vi "Untitled 5.vi"() -> ()   [LabVIEW 2015]
uses:
  <vilib>/Utility/Data Type/Type Definitions/Data Type.ctl
  <vilib>/Utility/Data Type/Type Definitions/Memory Info.ctl
  <vilib>/Utility/Data Type/Type Definitions/Memory Type.ctl
  <vilib>/Utility/Data Type/Type Definitions/Type Definition Info.ctl
  <vilib>/addons/msgpack/msgpack.lvlib
  <vilib>/Utility/Data Type/NI_Data Type.lvlib
  msgpackalt.dll
panel:
  out "dimension size":i32=3
  out "unsigned byte array 3":u8[](array[numeric]) format="%x"
  out "Type Definition Info":T1
  out "Array Lengths":T2[](array[typedef])
  out "Type 2":T4
  out "Type":T4
  out "data string 2":string
  out "Size(s)":u32[](array[numeric]) format="%x"
  out "data string":string
  out "unsigned byte array 2":u8[](array[numeric])
  out "unsigned byte array":u8[](array[numeric]) format="%x"
  out "size(s) 2":i32
  out "size(s)":i32 format="%x"
  out "data 2":variant[][][](array[variant])
  out "x-y":u32
  out "x = y?":bool
  out "data":string
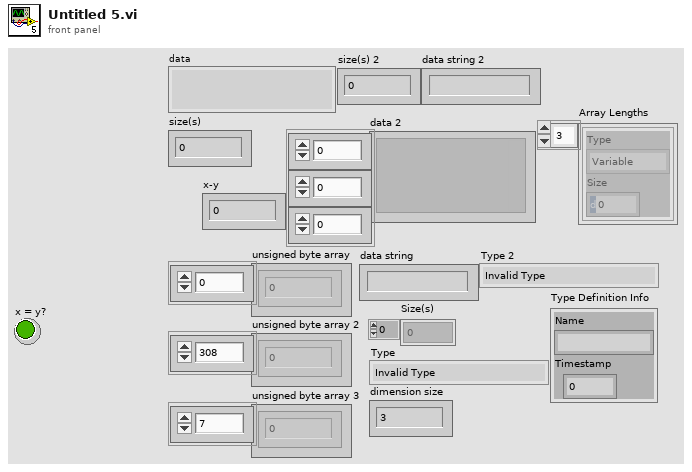
[diagram p1: front panel]
types:
  T1 = typedef "NI_Data Type.lvlib/Type Definition Info.ctl" = cluster{"Name":string, "Timestamp":u32}
  T2 = typedef "NI_Data Type.lvlib/Memory Info.ctl" = cluster{"Type":T3, "Size":u32}
  T3 = typedef "NI_Data Type.lvlib/Memory Type.ctl" = enum16{"Variable", "Fixed", "Bounded"}
  T4 = typedef "NI_Data Type.lvlib/Data Type.ctl" = enum8{"Invalid Type", "Void", "I8", "I16", "I32", "I64", "U8", "U16", "U32", "U64", "Single Float", "Double Float", "Extended Float", "Single Complex", "Double Complex", "Extended Complex", "Enum U8", "Enum U16", "Enum U32", "Enum U64", "Single Float With Unit", "Double Float With Unit", "Extended Float With Unit", "Single Complex with Unit", "Double Complex with Unit", "Extended Complex with Unit", "Boolean", "String", "Path", "Picture", "Tag", "Array", "Cluster", "Variant", "LV Variant", "Waveform", "Timestamp", "Digital Waveform", "Digital Data", "ExpressData", "Refnum", "External Data", "VI", "Poly VI", "LabVIEW Class Instance", "Fixed Point"}
  T5 = enum16{"big-endian, network order", "native, host order", "little-endian"}
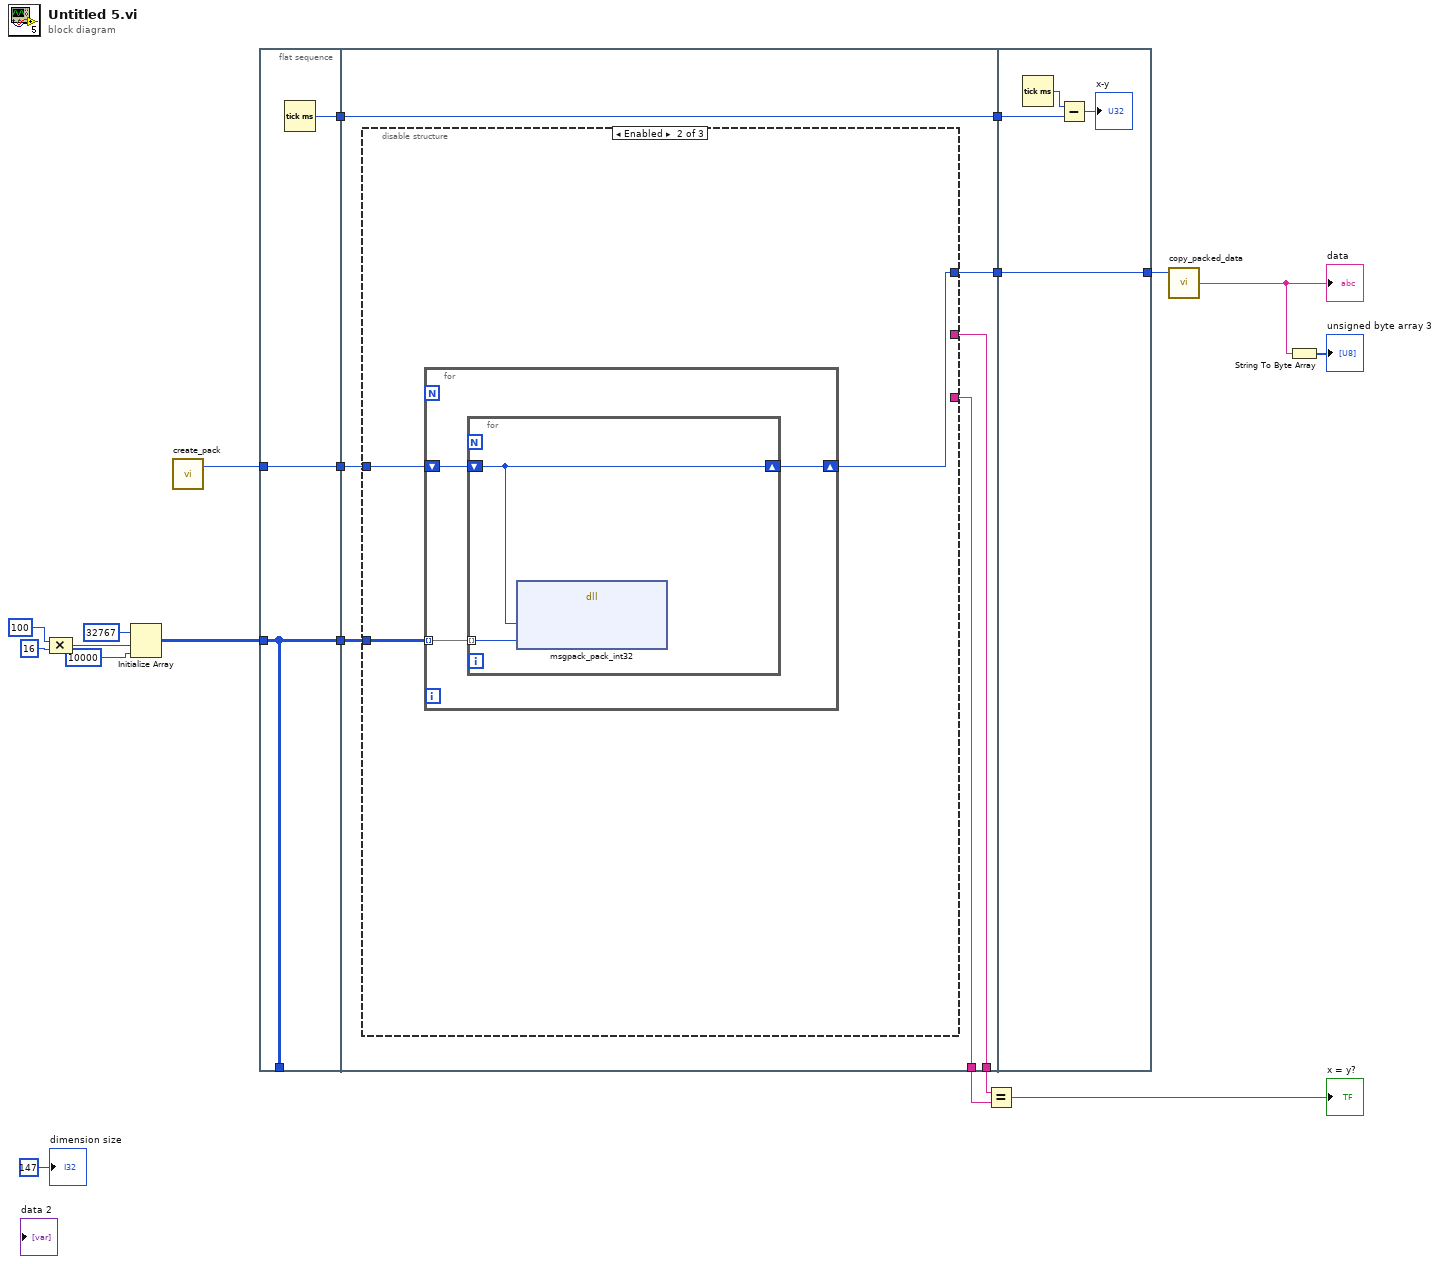
[diagram p0: block diagram]
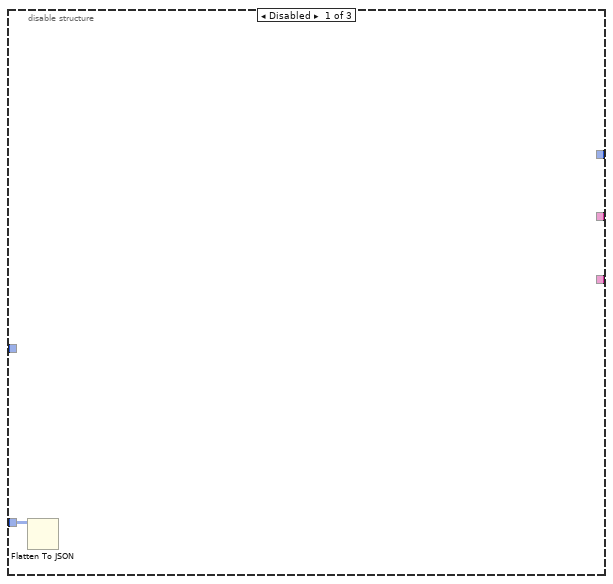
[diagram p2: hidden frame]
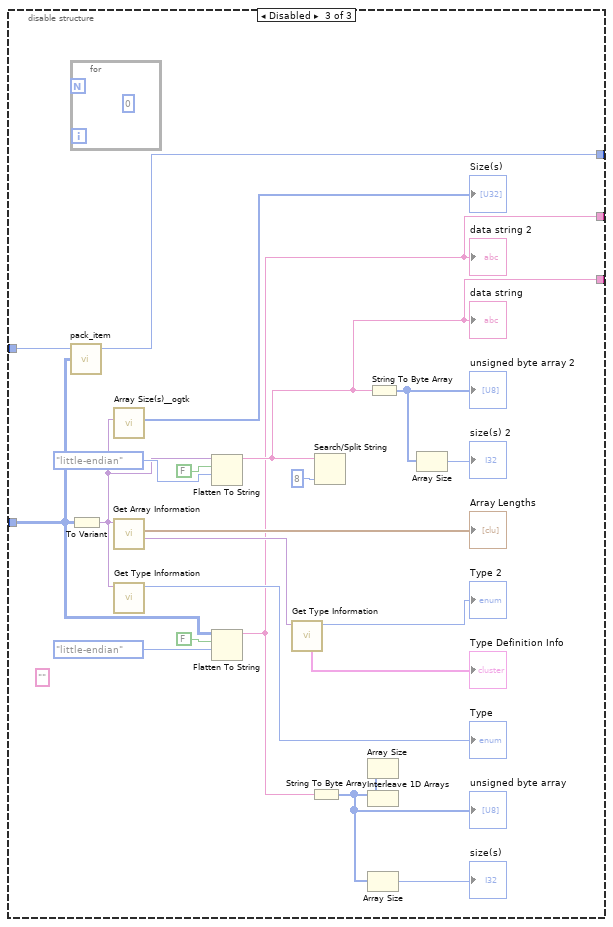
[diagram p3: hidden frame]
diagram:
  n1 = Compound Arithmetic op=MULTIPLY(100 ("dimension size"), 16 ("dimension size")) -> (w9:i32)
  n2 = Initialize Array(i16 32767 ("element"), w9, 10000 ("dimension size")) -> (w11:i16[][])
  n3 = call <vilib>:"create_pack.vi"() -> ("p"=w18:u64)  [unwired: 2 in, 1 out]
  n4 = flat-sequence {
    tunnel: w18 -> [w22]
    tunnel: [w22] -> w15
    tunnel: [w21] -> w14
    tunnel: [w20] -> w12
    tunnel: w11 -> [w20]
    tunnel: [w20] -> _
    tunnel: [w27] -> w16
    tunnel: w15 -> [w28]
    tunnel: w14 -> [w26]
    tunnel: [w26] -> w13
    tunnel: w12 -> [w25]
    tunnel: [w24] -> w8
    tunnel: [w23] -> w7
    tunnel: [w63] -> w17
    tunnel: w16 -> [w63]
    tunnel: w13 -> [w61]
    frame #0 {
      n5 = Tick Count (ms)() -> (millisecond timer value=w21:u32)
    }
    frame #1 {
      n6 = disable-structure shown="Enabled" {
        disable-tunnel: w28 -> [_ w32 w50]
        disable-tunnel: [_ w31 w48] -> w27
        disable-tunnel: w25 -> [w29 w30 w49]
        disable-tunnel: [_ _ w40] -> w24
        disable-tunnel: [_ _ w52] -> w23
        frame Disabled {
          n7 = Flatten To JSON(anything=w29) -> ()  [unwired: 2 in, 2 out]
        }
        frame Enabled {
          n8 = for {
            tunnel: w30 -> [w33] mode=indexing
            shift-right: [w34] -> w31
            shift-left: w32 -> [w35]
            n9 = for {
              tunnel: w33 -> [w37] mode=indexing
              shift-right: [w36] -> w34
              shift-left: w35 -> [w36]
              n10 = dll-call lib="S:/msgpack-lv/msgpackalt.dll" fn="msgpack_pack_int32"("p"=w36, "x"=w37) -> ()  [unwired: 6 in, 2 out]
            }
          }
        }
        frame Disabled {
          (unwired) "" ("data string")
          n11 = for {
            (unwired) u8 0
          }
          n12 = call <vilib>:"pack_item.vi"("x"=w49, "p"=w50) -> ("p out"=w48:u64)  [unwired: 2 in, 1 out]
          n13 = To Variant(anything=w49) -> (Variant=w46:variant)
          n14 = call <userlib>:"Array Size(s)__ogtk.vi"("Array"=w46) -> ("Size(s)"=→"Size(s)":u32[])  [unwired: 8 in, 2 out]
          n15 = call <vilib>:"Get Array Information.vi"("Variant"=w46) -> ("Array Element Data Type"=w44:variant, "Array Lengths"=→"Array Lengths":T2[])  [unwired: 7 in, 2 out]
          n16 = call <vilib>:"Get Type Information.vi"("Variant"=w46) -> ("Type"=→"Type":T4)  [unwired: 6 in, 4 out]
          n17 = Flatten To String(anything=w46, prepend array or string size? (T)=FALSE, byte order (0:big-endian, network order)=T5."little-endian") -> (data string=w52:string)  [unwired: 1 in, 2 out]
          "data string" <- w52
          n18 = Flatten To String(anything=w49, prepend array or string size? (T)=FALSE, byte order (0:big-endian, network order)=T5."little-endian") -> (data string=w40:string)  [unwired: 1 in, 2 out]
          "data string 2" <- w40
          n19 = call <vilib>:"Get Type Information.vi"("Variant"=w44) -> ("Type"=→"Type 2":T4, "Type Definition Info"=→"Type Definition Info":T1)  [unwired: 6 in, 3 out]
          n20 = String To Byte Array(string=w40) -> (unsigned byte array=w39:u8[])
          "unsigned byte array" <- w39
          n21 = Search/Split String(string=w52, offset (0)=8) -> ()  [unwired: 1 in, 3 out]
          n22 = Interleave 1D Arrays(w39) -> (w38:u8[])  [unwired: 1 out]
          n23 = Array Size(array=w38) -> ()  [unwired: 1 out]
          n24 = Array Size(array=w39) -> (size(s)=→"size(s)":i32)
          n25 = String To Byte Array(string=w52) -> (unsigned byte array=w57:u8[])
          "unsigned byte array 2" <- w57
          n26 = Array Size(array=w57) -> (size(s)=→"size(s) 2":i32)
        }
      }
    }
    frame #2 {
      n27 = Tick Count (ms)() -> (millisecond timer value=w62:u32)
      n28 = Subtract(x=w62, y=w61) -> (x-y=→"x-y":u32)
    }
  }
  n29 = Equal?(x=w8, y=w7) -> (x = y?=→"x = y?":bool)
  n30 = call <vilib>:"copy_packed_data.vi"("p"=w17) -> ("data"=w5:string)  [unwired: 2 in, 2 out]
  "data" <- w5
  n31 = String To Byte Array(string=w5) -> (unsigned byte array=→"unsigned byte array 3":u8[])
  "dimension size" <- 147
